vi "write_log_spike_data.vi"(8 "error in (no error)":errorcluster, 10 "Received Data 2":dbl, 11 "Log File in":refnum<k34>) -> (0 "error out":errorcluster, 3 "Log File out":refnum<k34>)   [LabVIEW 2017]
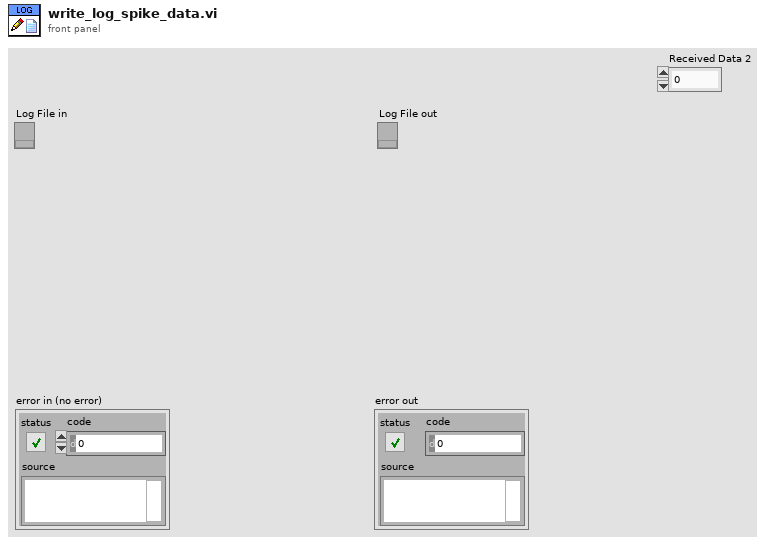
[diagram p1: front panel]
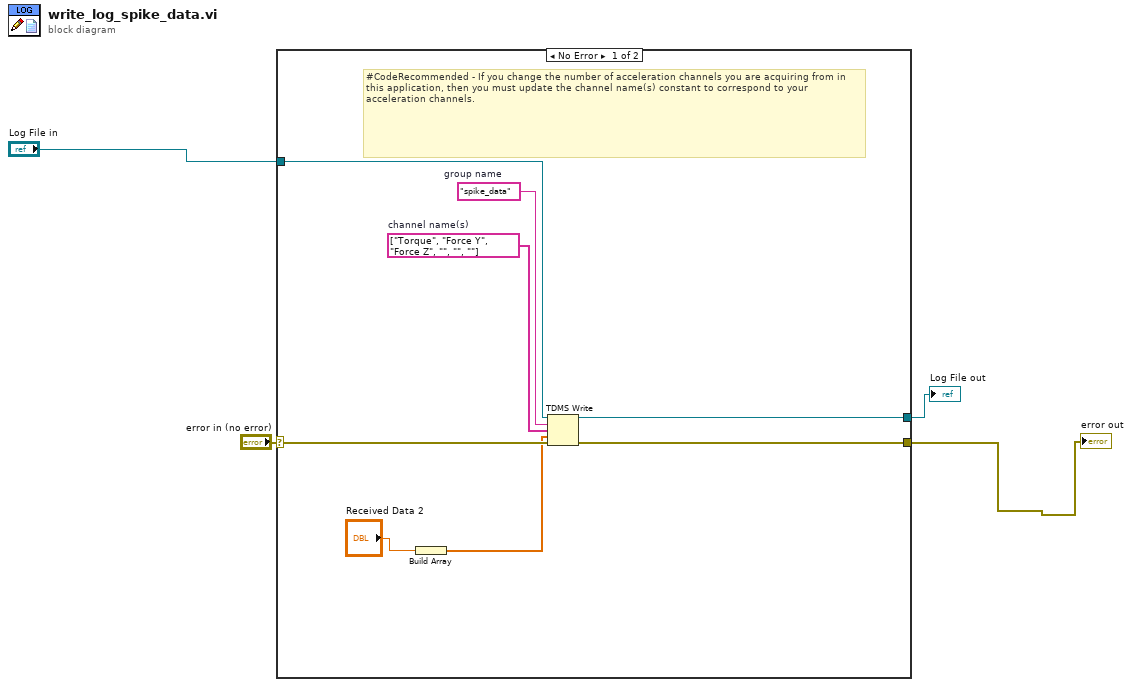
[diagram p0: block diagram]
diagram:
  n1 = case shown="No Error" "error in (no error)" {
    selector: "error in (no error)" -> [w8 w13]
    tunnel: "Log File in" -> [w10 w14]
    tunnel: [w9 w14] -> w3
    tunnel: [w7 w13] -> w1
    frame No Error {
      w11 = string[] ["Torque", "Force Y", "Force Z", "", "", ""]  # channel name(s)
      w12 = "spike_data"  # group name
      # "#CodeRecommended - If you change the number of acceleration channels you are acquiring from in this application, then you must update the channel name(s) constant to correspond to your acceleration channels."
      n2 = Build Array("Received Data 2") -> (w5:dbl[])
      n3 = TDMS Write(0:w10, 5:w12, 7:w11, 9:w5, 11:w8) -> (4:w9:refnum<k34>, 15:w7:errorcluster)  [unwired: 1 in, 2 out]
    }
    frame Error {
    }
  }
  "Log File out" <- w3
  "error out" <- w1
